vi "Request Data.vi"(4 "Ignore Past Updates? (F)":bool, 5 "Return Priority (Normal)":T2=enum."Normal", 6 "Value Changes Only? (T)":bool=TRUE, 7 "Activate Immediately? (T)":bool=TRUE, 8 "error in (no error)":errorcluster, 9 "Data Type":variant, 10 "Datum Name":string, 11 "IObserver in":refnum<class "IObserver.lvclass">) -> (0 "error out":errorcluster, 2 "Subscription Policy":T1, 3 "IObserver out":refnum<class "IObserver.lvclass">)   [LabVIEW 2017, in "IObserver.lvlib" / "IObserver.lvclass"]
doc: "<License>\nCopyright © 2017 Composed Systems, LLC | All rights reserved\nwww.composed.io\n\nAuthor: Ethan Stern <ethan.stern@composed.io>\n\nThis software is provided \"AS IS\" WITHOUT WARRANTIES, either express or implied, AND IS FOR EDUCATIONAL PURPOSES ONLY.\n</License>"
uses:
  IObserver.lvclass
  C:/Program Files (x86)/National Instruments/LabVIEW 2017/vi.lib/ActorFramework/Actor/Actor.lvclass
  <vilib>/ActorFramework/Message Enqueuer/Message Priority.ctl
  IMediator/ISubscriptionPolicy/ISubscriptionPolicy Reference.ctl
  IMediator/ISubscriptionPolicy/ISubscriptionPolicy.lvclass
  <vilib>/ActorFramework/Actor/Actor.lvclass/Actor.ctl
  <vilib>/ActorFramework/Message Enqueuer/Message Enqueuer.lvclass/Message Enqueuer.ctl
  SubscriptionPolicy/BasicSubscription/BasicSubscription.lvclass/BasicSubscription.ctl
  SubscriptionPolicy/ValueChangeSubscription/ValueChangeSubscription.lvclass/ValueChangeSubscription.ctl
  IMediator/SubscriptionRequest/SubscriptionRequest.lvclass/SubscriptionRequest.ctl
  IObserver Messages/Subscribe Msg/Subscribe Msg.lvclass/Subscribe Msg.ctl
  <vilib>/ActorFramework/Message Enqueuer/Init from Existing Queue.vi
  <vilib>/ActorFramework/Message Enqueuer/Enqueue.vi
  SubscriptionPolicy/BasicSubscription/BasicSubscription.lvclass
  C:/Git/mva-framework/Framework/IMediator/ISubscriptionPolicy/ISubscriptionPolicy.lvclass
  SubscriptionPolicy/ValueChangeSubscription/ValueChangeSubscription.lvclass
  ActorDataBinding/ActorDataBinding.lvclass
  C:/Git/mva-framework/Framework/IMediator/ITransport/ITransport.lvclass
  IObserver Messages/Subscribe Msg/Subscribe Msg.lvclass
  C:/Program Files (x86)/National Instruments/LabVIEW 2017/vi.lib/ActorFramework/Message/Message.lvclass
  <vilib>/ActorFramework/Message Priority Queue/Priority Enqueue.vi
  IMediator/SubscriptionRequest/SubscriptionRequest.lvclass
  <vilib>/ActorFramework/Message Enqueuer/Message Enqueuer.lvclass
  <vilib>/ActorFramework/Actor/Actor.lvclass
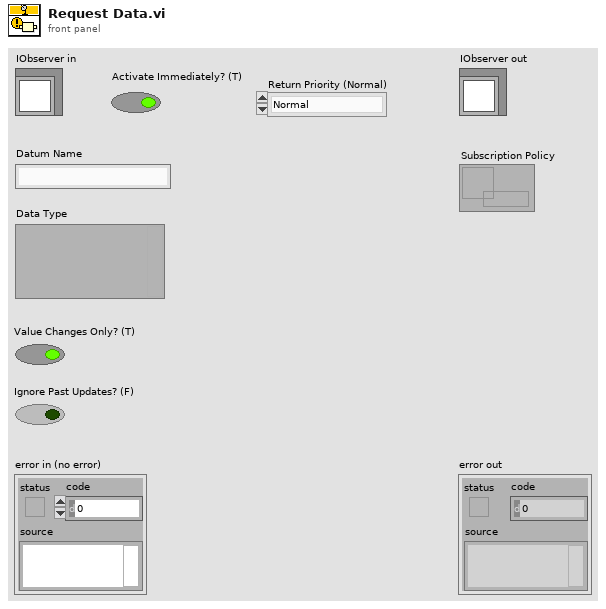
[diagram p1: front panel]
types:
  T1 = typedef "IMediator.lvlib/ISubscriptionPolicy.lvclass/ISubscriptionPolicy Reference.ctl" = refnum<data-value>
  T2 = typedef "Actor Framework.lvlib/Message Enqueuer.lvclass/Message Priority.ctl" = enum16{"Low", "Normal", "High"}
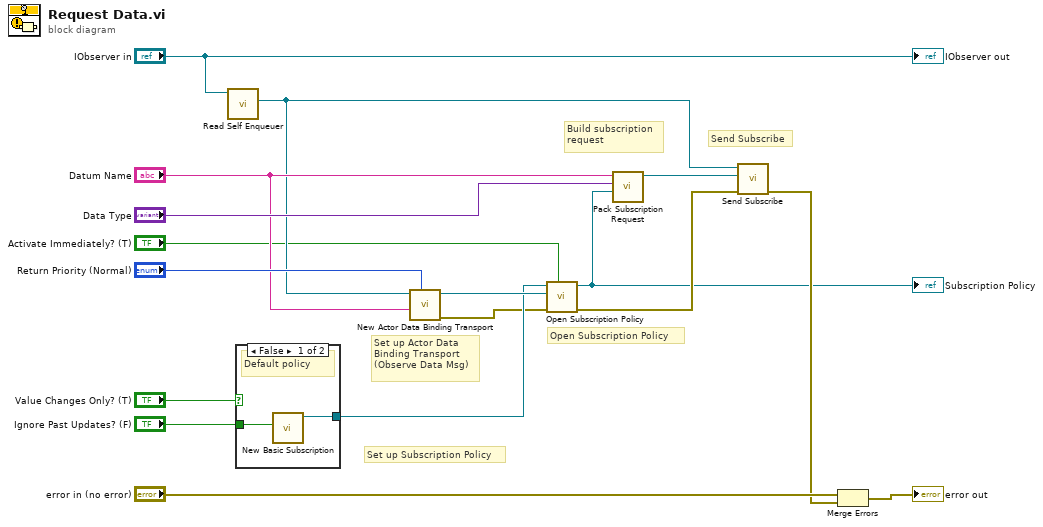
[diagram p0: block diagram]
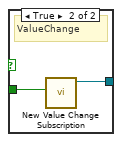
[diagram p2: hidden frame]
diagram:
  # "Open Subscription Policy"
  # "Set up Subscription Policy"
  # "Send Subscribe"
  # "Build subscription\nrequest"
  # "Set up Actor Data\nBinding Transport\n(Observe Data Msg)"
  n1 = call <vilib>:"Read Self Enqueuer.vi"("Actor"="IObserver in") -> ("Self Enqueuer"=w3:refnum<class "Message Enqueuer.lvclass">)  [unwired: 10 in]
  n2 = case shown="False" "Value Changes Only? (T)" {
    tunnel: "Ignore Past Updates? (F)" -> [w18 w21]
    tunnel: [w19 w20] -> w11
    frame False {
      # "Default policy"
      n3 = call "New Basic Subscription.vi"("Ignore Past Updates? (F)"=w18) -> ("BasicSubscription Out"=w19:refnum<class "BasicSubscription.lvclass">)  [unwired: 10 in]
    }
    frame True {
      # "ValueChange"
      n4 = call "New Value Change Subscription.vi"("Ignore Past Updates? (F)"=w21) -> ("ValueChangeSubscription Out"=w20:refnum<class "ValueChangeSubscription.lvclass">)  [unwired: 10 in]
    }
  }
  n5 = call "New Actor Data Binding Transport.vi"("Priority (Normal)"="Return Priority (Normal)", "Datum Return Name"="Datum Name", "IObserver"=w3) -> ("error out"=w8:errorcluster, "ActorDataBinding out"=w14:refnum<class "ActorDataBinding.lvclass">)  [unwired: 7 in]
  n6 = call "Open Subscription Policy.vi"("Activate? (T)"="Activate Immediately? (T)", "error in (no error)"=w8, "Transport"=w14, "SubscriptionPolicy"=w11) -> ("error out"=w5:errorcluster, "Subscription Policy"=w1:T1)  [unwired: 6 in]
  "Subscription Policy" <- w1
  n7 = call "Pack Subscription Request.vi"("Subscription Policy"=w1, "Type"="Data Type", "Datum Name"="Datum Name") -> ("SubscriptionRequest"=w6:refnum<class "SubscriptionRequest.lvclass">)  [unwired: 8 in]
  n8 = call "Send Subscribe.vi"("error in (no error)"=w5, "SubscriptionRequest"=w6, "Message Enqueuer"=w3) -> ("error out"=w4:errorcluster)  [unwired: 7 in, 1 out]
  n9 = Merge Errors("error in (no error)", w4) -> (→"error out":errorcluster)
  "IObserver out" <- "IObserver in"
